vi "add_AccelStamped_roslv.vi"(5 "Accel":T1, 6 "Stamp":cluster{"frame_id":string, "reset seq?":bool}, 7 "msg in":string) -> (3 "msg out":string)   [LabVIEW 2014]
doc: "Flattens a stamped acceleration into a message"
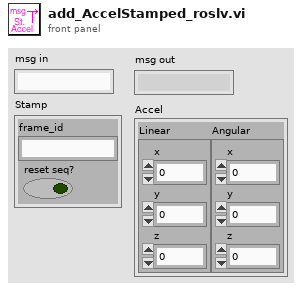
[diagram p1: front panel]
types:
  T1 = cluster{"Linear":cluster{"x":dbl, "y":dbl, "z":dbl}, "Angular":cluster{"x":dbl, "y":dbl, "z":dbl}}
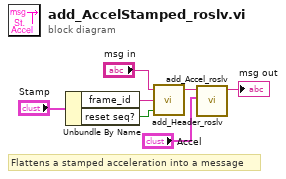
[diagram p0: block diagram]
diagram:
  # "Flattens a stamped acceleration into a message"
  n1 = Unbundle By Name("Stamp") -> ("frame_id"=w5:string, "reset seq?"=w4:bool)
  n2 = call "add_Header_roslv.vi"("reset seq?"=w4, "frame_id"=w5, "msg in"="msg in") -> ("msg out"=w3:string)  [unwired: 2 in]
  n3 = call "add_Accel_roslv.vi"("Accel"="Accel", "msg in"=w3) -> ("msg out"=→"msg out":string)  [unwired: 5 in]
